vi "RT_TVA_Plant (SubVI).vi"(8 "TVA_b(i-2)":dbl[](array[numeric]), 9 "TVA_b(i-1)":dbl[](array[numeric]), 10 "TVA_cmd (i-2) [rad]":dbl[](array[numeric]), 11 "TVA_cmd (i-1) [rad]":dbl[](array[numeric])) -> (3 "TVA_b":dbl[](array[numeric]))   [LabVIEW 2017]
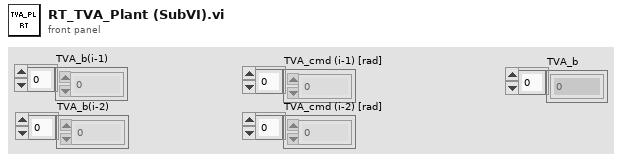
[diagram p1: front panel]
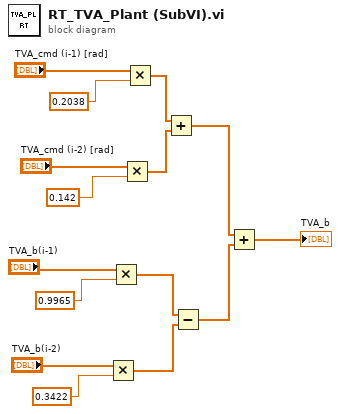
[diagram p0: block diagram]
diagram:
  n1 = Multiply(x="TVA_b(i-2)", y=0.3422) -> (x*y=w10:dbl[])
  n2 = Multiply(x="TVA_b(i-1)", y=0.9965) -> (x*y=w11:dbl[])
  n3 = Multiply(x="TVA_cmd (i-2) [rad]", y=0.142) -> (x*y=w4:dbl[])
  n4 = Multiply(x="TVA_cmd (i-1) [rad]", y=0.2038) -> (x*y=w5:dbl[])
  n5 = Add(x=w5, y=w4) -> (x+y=w3:dbl[])
  n6 = Subtract(x=w11, y=w10) -> (x-y=w2:dbl[])
  n7 = Add(x=w3, y=w2) -> (x+y=→"TVA_b":dbl[])
